vi "onStart.vi"(8 "error in (no error)":errorcluster, 11 "SMO":refnum<class "SMO.lvclass">) -> (0 "error out":errorcluster, 3 "SMO out":refnum<class "SMO.lvclass">)   [LabVIEW 2013, in "SMO.lvclass"]
uses:
  SMO.lvclass
  Dependency/Dependency.lvclass/Dependency.ctl
  Dependency/Dependency.lvclass
panel:
  # "For instructions on how to use the JKI State Machine Objects, examples and video tutorials, visit:\nhttp://jki.net/state-machine-objects/\n\nJKI State Machine Objects™\nhttp://jki.net/state-machine-objects/\nCopyright (C) 2005-2015, JKI <info@jki.net>\nALL RIGHTS RESERVED"
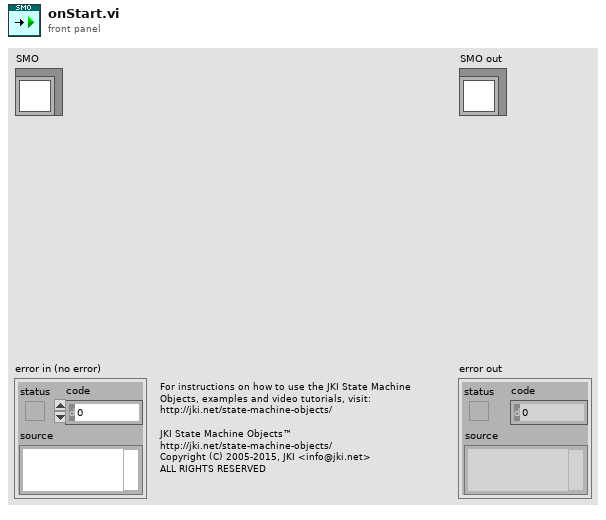
[diagram p1: front panel]
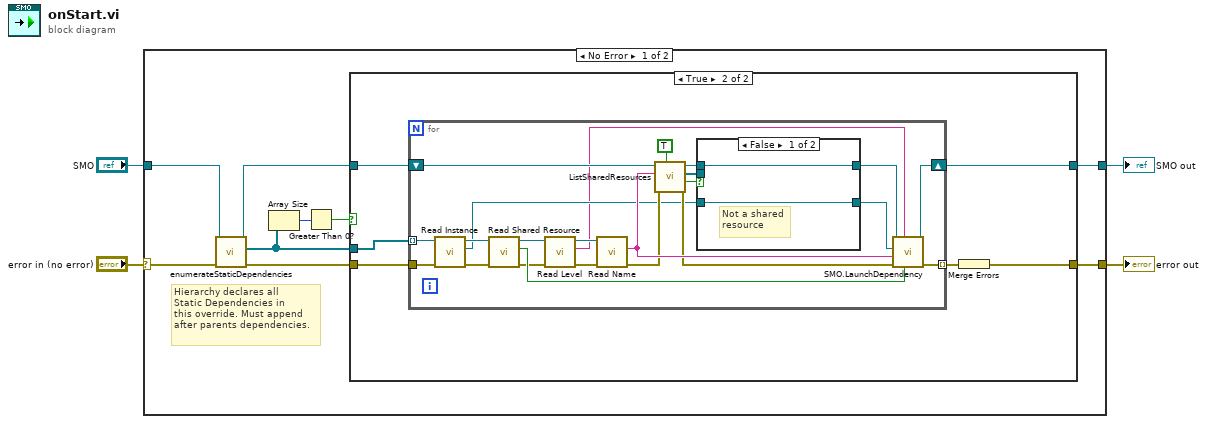
[diagram p0: block diagram]
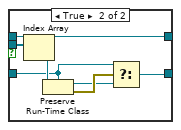
[diagram p3: hidden frame]
diagram:
  n1 = case shown="No Error" "error in (no error)" {
    selector: "error in (no error)" -> [w7 w55]
    tunnel: [w12 w55] -> w3
    tunnel: [w13 w54] -> w1
    tunnel: "SMO" -> [w9 w54]
    frame No Error {
      # "Hierarchy declares all\nStatic Dependencies in\nthis override. Must append\nafter parents dependencies."
      n2 = call-dynamic "enumerateStaticDependencies.vi"("error in (no error)"=w7, "SMO"=w9) -> ("error out"=w6:errorcluster, "Static Dependencies"=w5:refnum<class "Dependency.lvclass">[], "SMO out"=w8:refnum<class "SMO.lvclass">)  [unwired: 7 in]
      n3 = Array Size(array=w5) -> (size(s)=w11:i32)
      n4 = Greater Than 0?(x=w11) -> (x > 0?=w10:bool)
      n5 = case shown="True" w10 {
        tunnel: w5 -> [_ w21]
        tunnel: w8 -> [w15 w17]
        tunnel: w6 -> [w14 w20]
        tunnel: [w15 w19] -> w13
        tunnel: [w14 w18] -> w12
        frame False {
        }
        frame True {
          n6 = for {
            tunnel: w21 -> [w44] mode=indexing
            tunnel: w20 -> [w43]
            tunnel: [w42] -> w16 mode=indexing
            shift-right: [w41] -> w19
            shift-left: w17 -> [w37]
            n7 = call "Read Instance.vi"("error in (no error)"=w43, "Dependency in"=w44) -> ("error out"=w39:errorcluster, "SMO.lvclass"=w27:refnum<class "SMO.lvclass">, "Dependency out"=w40:refnum<class "Dependency.lvclass">)  [unwired: 7 in]
            n8 = call "Read Shared Resource.vi"("error in (no error)"=w39, "Dependency in"=w40) -> ("error out"=w26:errorcluster, "Shared Resource"=w38:bool, "Dependency out"=w25:refnum<class "Dependency.lvclass">)  [unwired: 7 in]
            n9 = call "Read Level.vi"("error in (no error)"=w26, "Dependency in"=w25) -> ("error out"=w23:errorcluster, "Level"=w22:string, "Dependency out"=w24:refnum<class "Dependency.lvclass">)  [unwired: 7 in]
            n10 = call "Read Name.vi"("error in (no error)"=w23, "Dependency in"=w24) -> ("error out"=w34:errorcluster, "Name"=w35:string)  [unwired: 7 in, 1 out]
            n11 = call "ListSharedResources.vi"("exact name? (F: regex)"=TRUE, "error in (no error)"=w34, "Filter (regex|name)"=w35, "SMO in"=w37) -> ("error out"=w33:errorcluster, "resources found?"=w29:bool, "Shared Resources"=w32:refnum<class "SMO.lvclass">[], "SMO out"=w31:refnum<class "SMO.lvclass">)  [unwired: 4 in]
            n12 = case shown="False" w29 {
              tunnel: w32 -> [_ w53]
              tunnel: w31 -> [w46 w52]
              tunnel: [w46 w52] -> w30
              tunnel: [w45 w48] -> w28
              tunnel: w27 -> [w45 w47]
              frame False {
                # "Not a shared\nresource"
              }
              frame True {
                n13 = Index Array(array=w53) -> (element=w51:refnum<class "SMO.lvclass">)  [unwired: 1 in]
                n14 = Preserve Run-Time Class(object in=w51, 2:w47) -> (object out=w49:refnum<class "SMO.lvclass">, error out=w50:errorcluster)  [unwired: 1 in]
                n15 = Select(t=w47, s=w50, f=w49) -> (s? t:f=w48:refnum<class "SMO.lvclass">)
              }
            }
            n16 = call "SMO.LaunchDependency.vi"("Shared Resource"=w38, "Level"=w22, "error in (no error)"=w33, "Dependency Name"=w35, "Dependency Type"=w28, "SMO in"=w30) -> ("error out"=w42:errorcluster, "SMO out"=w41:refnum<class "SMO.lvclass">)  [unwired: 3 in, 1 out]
          }
          n17 = Merge Errors(w16) -> (w18:errorcluster)
        }
      }
    }
    frame Error {
    }
  }
  "error out" <- w3
  "SMO out" <- w1
